vi "Panel-AlignRasterPI.vi"() -> ()   [LabVIEW 2009]
uses:
  Instance           6 29Saved   RasterPI-Continuous2D .vi
  Instance           9 29Saved   RasterPI-Continuous2D .vi
panel:
  out "Bary Y":dbl format="%.2f"
  out "Bary X":dbl format="%.2f"
  in  "PI Number":enum16{"1", "2"}(ring)=enum."2"
  out "Graphe d'intensité":dbl[][](graph)=[[283.6564867337676, 290.6564867337676, 297.6564867337676, 332.6564867337676, 288.65648673376757, 376.6564867337676, 274.6564867337676], [455.6564867337676, 284.6564867337676, 249.6564867337676, 354.6564867337676, 368.6564867337676, 310.6564867337676, 281.6564867337676], [381.6564867337676, 224.6564867337676, 377.6564867337676, 235.65648673376762, 338.6564867337676, 286.6564867337676, 340.6564867337676], [397.6564867337676, 278.6564867337676, 289.6564867337676, 172.65648673376762, 333.6564867337676, 267.6564867337676, 248.65648673376762], [315.6564867337676, 226.65648673376762, 302.6564867337676, 220.65648673376762, 369.6564867337676, 243.6564867337676, 323.6564867337676], [338.6564867337676, 207.65648673376762, 398.6564867337676, 271.6564867337676, 256.6564867337676, 299.6564867337676, 283.6564867337676], [331.6564867337676, 251.65648673376762, 370.6564867337676, 324.6564867337676, 268.6564867337676, 281.6564867337676, 263.6564867337676]]
  in  "Integration time":dbl=1.0
  in  "Steps":i32=7
  in  "Step size":i32=2000
  out "Graphe":dbl[](graph)=[331.6564867337676, 251.65648673376762, 370.6564867337676, 324.6564867337676, 268.6564867337676, 281.6564867337676, 263.6564867337676]
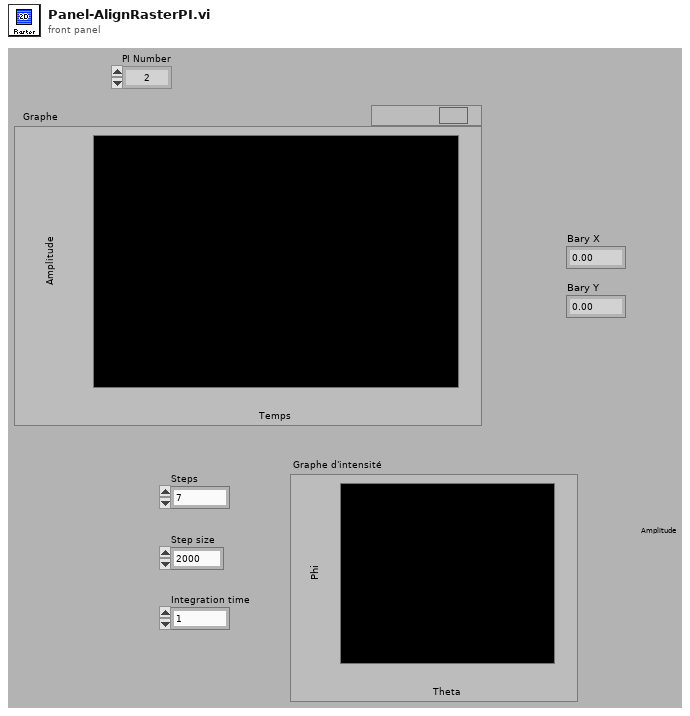
[diagram p1: front panel]
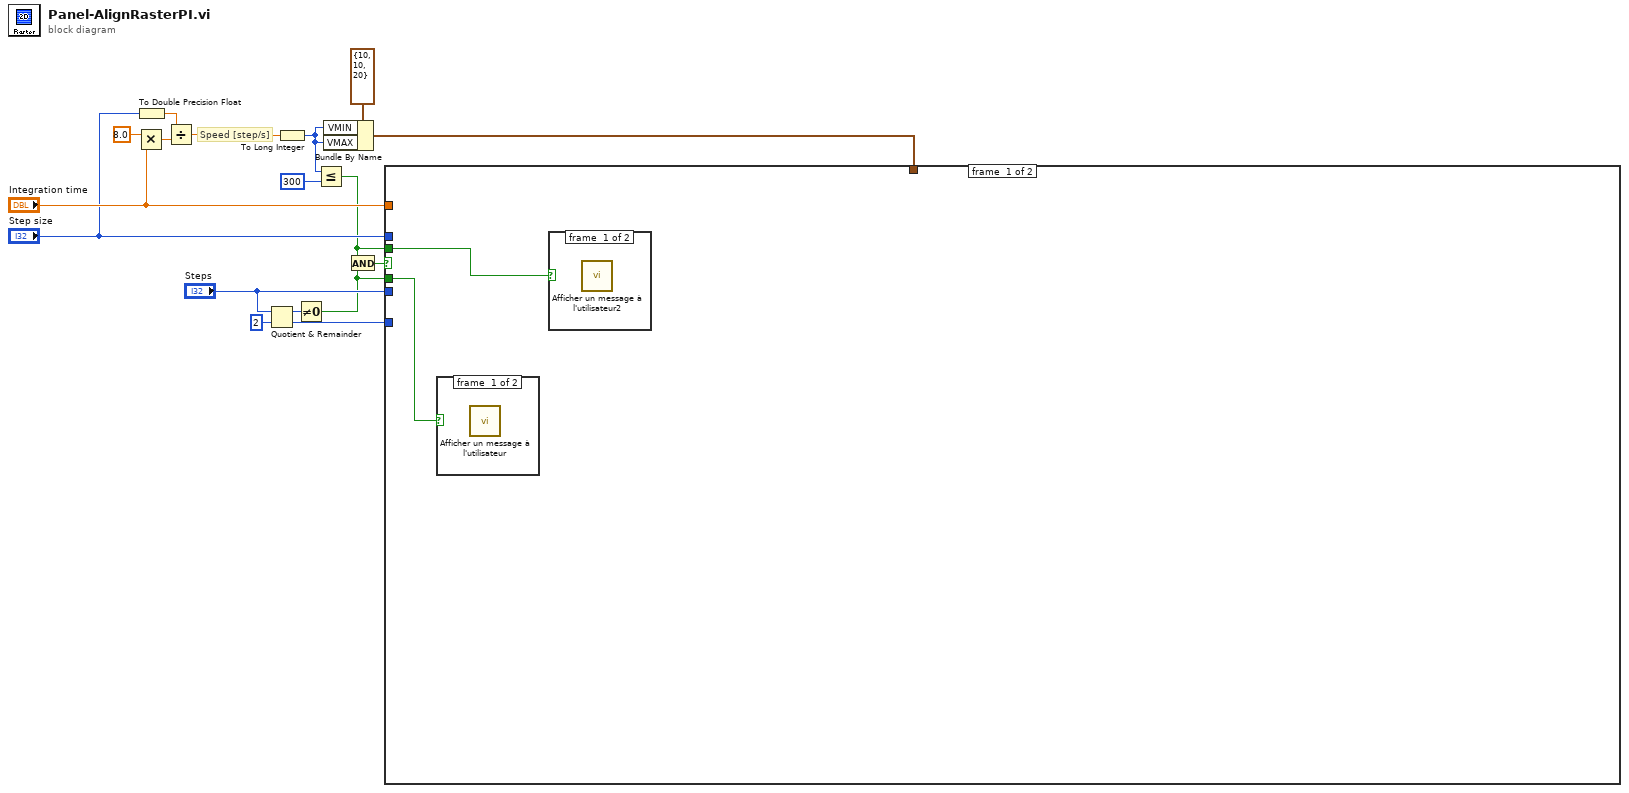
[diagram p0: block diagram]
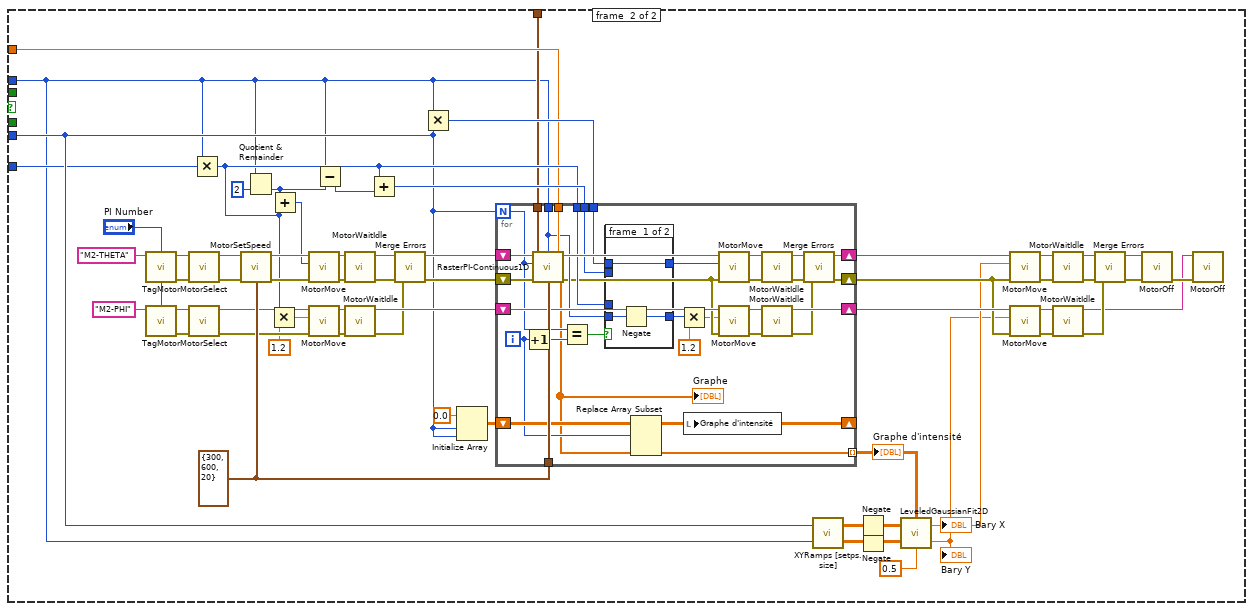
[diagram p4: hidden frame]
diagram:
  # "Speed [step/s]"
  n1 = Multiply(x=8.0 ("valeur"), y="Integration time") -> (x*y=w10:dbl)
  n2 = To Double Precision Float(number="Step size") -> (double precision float=w13:dbl)
  n3 = Divide(x=w13, y=w10) -> (x/y=w11:dbl)
  n4 = Quotient & Remainder(x="Steps", y=2) -> (x-y*floor(x/y)=w14:i32, floor(x/y)=w16:i32)
  n5 = To Long Integer(number=w11) -> (32bit integer=w6:i32)
  n6 = Not Equal To 0?(x=w14) -> (x != 0?=w1:bool)
  n7 = Less Or Equal?(x=w6, y=300) -> (x <= y?=w2:bool)
  n8 = Bundle By Name(cluster=cluster{"VMIN":i32, "VMAX":i32, "ACC":i32} {"VMIN"=10, "VMAX"=10, "ACC"=20} ("Param"), "VMIN"=w6, "VMAX"=w6) -> (w4:cluster{"VMIN":i32, "VMAX":i32, "ACC":i32})
  n9 = And(x=w2, y=w1) -> (x .and. y?=w3:bool)
  n10 = case shown="True" w3 {
    tunnel: w16 -> [_ w41]
    tunnel: "Steps" -> [_ w42]
    tunnel: "Integration time" -> [_ w44]
    tunnel: "Step size" -> [_ w37]
    tunnel: w4 -> [_ w43]
    tunnel: w2 -> [w18 _]
    tunnel: w1 -> [w19 _]
    frame #0 {
      n11 = case shown="False" w19 {
        frame #0 {
          n12 = call "Afficher un message à l'utilisateur"() -> ()  [unwired: 3 in, 9 out]
        }
        frame #1 {
        }
      }
      n13 = case shown="False" w18 {
        frame #0 {
          n14 = call "Afficher un message à l'utilisateur2"() -> ()  [unwired: 3 in, 9 out]
        }
        frame #1 {
        }
      }
    }
    frame #1 {
      w72 = cluster{"VMIN":i32, "VMAX":i32, "ACC":i32} {"VMIN"=300, "VMAX"=600, "ACC"=20} ("Param")
      n15 = call "TagMotor.vi"("PI Number"="PI Number", "Motor"="M2-THETA") -> ("Tagged Motor"=w48:string, "error out"=w47:errorcluster)  [unwired: 1 in, 5 out]
      n16 = call "TagMotor.vi"("PI Number"="PI Number", "Motor"="M2-PHI") -> ("Tagged Motor"=w50:string, "error out"=w49:errorcluster)  [unwired: 1 in, 5 out]
      n17 = call "MotorSelect.vi"("Motor"=w48, "error in (no error)"=w47) -> ("Motor out"=w79:string, "error out"=w78:errorcluster)  [unwired: 6 out]
      n18 = call "MotorSelect.vi"("Motor"=w50, "error in (no error)"=w49) -> ("Motor out"=w68:string, "error out"=w69:errorcluster)  [unwired: 6 out]
      n19 = Multiply(x=w37, y=w41) -> (x*y=w53:i32)
      n20 = call "MotorSetSpeed.vi"("Param"=w72, "Motor"=w79, "error in (no error)"=w78) -> ("Motor out"=w77:string, "error out"=w76:errorcluster)  [unwired: 5 out]
      n21 = Quotient & Remainder(x=w37, y=2) -> (floor(x/y)=w57:i32)  [unwired: 1 out]
      n22 = Multiply(x=w53, y=1.2) -> (x*y=w54:dbl)
      n23 = Add(x=w57, y=w53) -> (x+y=w58:i32)
      n24 = call "MotorMove.vi"("Motor"=w77, "Movement"=w58, "error in (no error)"=w76) -> ("Motor out"=w74:string, "error out"=w75:errorcluster)  [unwired: 5 out]
      n25 = call "MotorMove.vi"("Motor"=w68, "Movement"=w54, "error in (no error)"=w69) -> ("Motor out"=w71:string, "error out"=w70:errorcluster)  [unwired: 5 out]
      n26 = Subtract(x=w37, y=w57) -> (x-y=w56:i32)
      n27 = call "MotorWaitIdle.vi"("Motor"=w74, "error in (no error)"=w75) -> ("Motor out"=w73:string, "error out"=w65:errorcluster)  [unwired: 6 out]
      n28 = call "MotorWaitIdle.vi"("Motor"=w71, "error in (no error)"=w70) -> ("Motor out"=w67:string, "error out"=w63:errorcluster)  [unwired: 6 out]
      n29 = Add(x=w53, y=w56) -> (x+y=w55:i32)
      n30 = call <vilib>:"Merge Errors.vi"("error in 3 (no error)"=w63, "error in 2 (no error)"=w65) -> ("error out"=w64:errorcluster)  [unwired: 2 in, 3 out]
      n31 = Multiply(x=w37, y=w42) -> (x*y=w66:i32)
      n32 = Initialize Array(0.0 ("élément"), w42, w42) -> (w60:dbl[][])
      n33 = for {
        N: w42 -> [w95]
        tunnel: w72 -> [w109]
        tunnel: w44 -> [w108]
        tunnel: w37 -> [w101]
        shift-right: [w99] -> w29
        shift-left: w67 -> [w102]
        shift-right: [w89] -> w28
        shift-left: w64 -> [w111]
        shift-right: [w100] -> w30
        shift-left: w73 -> [w110]
        tunnel: w66 -> [w97]
        tunnel: w53 -> [w93]
        shift-right: [w86] -> _
        shift-left: w60 -> [w88]
        tunnel: w55 -> [w85]
        tunnel: [w84] -> w38 mode=indexing
        tunnel: w43 -> [w80]
        i -> [w87]
        n34 = Increment(x=w87) -> (x+1=w96:i32)
        n35 = call "RasterPI-Continuous1D.vi"("Integration time"=w108, "Step size"=w101, "Motor in"=w110, "Steps"=w95, "Previous Speed"=w109, "Scan speed"=w80, "error in"=w111) -> ("Motor out"=w105:string, "Graphe"=w84:dbl[], "error in (no error)"=w92:errorcluster)
        "Graphe" <- w84
        n36 = Equal?(x=w95, y=w96) -> (x = y?=w94:bool)
        n37 = case shown="False" w94 {
          tunnel: w101 -> [w114 _]
          tunnel: [w113 w116] -> w82
          tunnel: [w112 w115] -> w98
          tunnel: w97 -> [w112 _]
          tunnel: w93 -> [_ w116]
          tunnel: w85 -> [_ w115]
          frame #0 {
            n38 = Negate(x=w114) -> (-x=w113:i32)
          }
          frame #1 {
          }
        }
        n39 = Replace Array Subset(array=w88, new element=w84, index (row)=w87) -> (w86:dbl[][])  [unwired: 1 in]
        n40 = Multiply(x=w82, y=1.2) -> (x*y=w81:dbl)
        n41 = local write "Graphe d'intensité"(w86) -> ()
        n42 = call "MotorMove.vi"("Motor"=w105, "Movement"=w98, "error in (no error)"=w92) -> ("Motor out"=w107:string, "error out"=w106:errorcluster)  [unwired: 5 out]
        n43 = call "MotorMove.vi"("Motor"=w102, "Movement"=w81, "error in (no error)"=w92) -> ("Motor out"=w103:string, "error out"=w104:errorcluster)  [unwired: 5 out]
        n44 = call "MotorWaitIdle.vi"("Motor"=w107, "error in (no error)"=w106) -> ("Motor out"=w100:string, "error out"=w91:errorcluster)  [unwired: 6 out]
        n45 = call "MotorWaitIdle.vi"("Motor"=w103, "error in (no error)"=w104) -> ("Motor out"=w99:string, "error out"=w90:errorcluster)  [unwired: 6 out]
        n46 = call <vilib>:"Merge Errors.vi"("error in 3 (no error)"=w90, "error in 2 (no error)"=w91) -> ("error out"=w89:errorcluster)  [unwired: 2 in, 3 out]
      }
      "Graphe d'intensité" <- w38
      n47 = call "XYRamps [setps.size].vi"("Step size"=w37, "Steps"=w42) -> ("Y"=w39:dbl[][], "X"=w40:dbl[][])
      n48 = Negate(x=w40) -> (-x=w22:dbl[][])
      n49 = Negate(x=w39) -> (-x=w21:dbl[][])
      n50 = call "LeveledGaussianFit2D.vi"("Coord Y"=w21, "Threshold"=0.5, "Coord X"=w22, "Image"=w38) -> ("Bary Y"=w23:dbl, "Bary X"=w24:dbl)
      "Bary X" <- w24
      "Bary Y" <- w23
      n51 = call "MotorMove.vi"("Motor"=w30, "Movement"=w24, "error in (no error)"=w28) -> ("Motor out"=w31:string, "error out"=w32:errorcluster)  [unwired: 5 out]
      n52 = call "MotorMove.vi"("Motor"=w29, "Movement"=w23, "error in (no error)"=w28) -> ("Motor out"=w34:string, "error out"=w33:errorcluster)  [unwired: 5 out]
      n53 = call "MotorWaitIdle.vi"("Motor"=w31, "error in (no error)"=w32) -> ("Motor out"=w26:string, "error out"=w35:errorcluster)  [unwired: 6 out]
      n54 = call "MotorWaitIdle.vi"("Motor"=w34, "error in (no error)"=w33) -> ("Motor out"=w25:string, "error out"=w36:errorcluster)  [unwired: 6 out]
      n55 = call <vilib>:"Merge Errors.vi"("error in 3 (no error)"=w36, "error in 2 (no error)"=w35) -> ("error out"=w27:errorcluster)  [unwired: 2 in, 3 out]
      n56 = call "MotorOff.vi"("Motor"=w26, "error in (no error)"=w27) -> ("error out"=w62:errorcluster)  [unwired: 7 out]
      n57 = call "MotorOff.vi"("Motor"=w25, "error in (no error)"=w62) -> ()  [unwired: 8 out]
    }
  }
